vi "Close.vi"(8 "error in (no error)":errorcluster, 11 "niPower in":refnum<class "NI DC Power.lvclass">) -> (0 "error out":errorcluster, 3 "niPower out":refnum<class "NI DC Power.lvclass">)   [LabVIEW 2025, in "Power Supply.lvlib" / "NI DC Power.lvclass"]
uses:
  NI DC Power.lvclass
  NI DC Power.lvclass/NI DC Power.ctl
  PS Instrument/Power Supply Instrument.lvclass
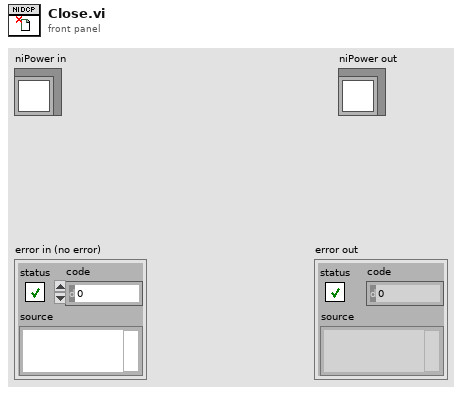
[diagram p1: front panel]
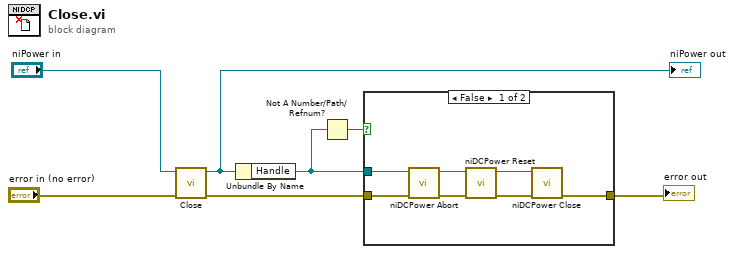
[diagram p0: block diagram]
diagram:
  n1 = call-parent "Close.vi"("error in (no error)"="error in (no error)", "Power Supply Instrument in"="niPower in") -> ("error out"=w3:errorcluster, "Power Supply Instrument out"=w1:refnum<class "NI DC Power.lvclass">)  [unwired: 8 in]
  "niPower out" <- w1
  n2 = Unbundle By Name(w1) -> ("Handle"=w5:refnum<k15>)
  n3 = Not A Number/Path/Refnum?(number/path/refnum=w5) -> (NaN/Path/Refnum?=w4:bool)
  n4 = case shown="False" w4 {
    tunnel: [w13 w15] -> w7
    tunnel: w3 -> [w11 w15]
    tunnel: w5 -> [w8 _]
    frame False {
      n5 = call <instrlib>:"niDCPower Abort.vi"("error in (no error)"=w11, "instrument handle"=w8) -> ("error out"=w9:errorcluster, "instrument handle out"=w10:refnum<k15>)  [unwired: 8 in]
      n6 = call <instrlib>:"niDCPower Reset.vi"("error in (no error)"=w9, "instrument handle"=w10) -> ("error out"=w14:errorcluster, "instrument handle out"=w12:refnum<k15>)  [unwired: 2 in, 6 out]
      n7 = call <instrlib>:"niDCPower Close.vi"("error in (no error)"=w14, "instrument handle"=w12) -> ("error out"=w13:errorcluster)  [unwired: 9 out]
    }
    frame True {
    }
  }
  "error out" <- w7
